vi "Unreachable.vi"   [LabVIEW 2018, in "GLog.lvlib" / "Utilities.lvlib"]
uses:
  Utilities.lvlib
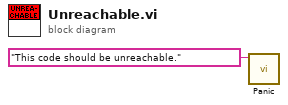
[diagram p0: block diagram]
diagram:
  n1 = call "Panic.vi"("message (\"\")"="This code should be unreachable." ("message (\"\")")) -> ()  [unwired: 11 in]
